vi "Initialize DAQDict Ref.vi"(8 "error in (no error)":errorcluster) -> (0 "error out":errorcluster, 3 "dCVT DAQDict out":T1)   [LabVIEW 2020, in "DAQDict.lvlib"]
uses:
  DAQDict.lvlib
  <vilib>/TELLC/Dynamic CVT API/TD Dynamic CVT DVR--ref.ctl
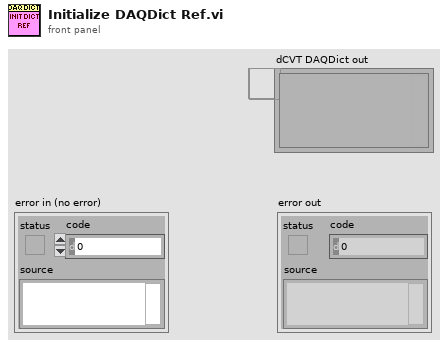
[diagram p1: front panel]
types:
  T1 = typedef "TD Dynamic CVT DVR--ref.ctl" = refnum<data-value>
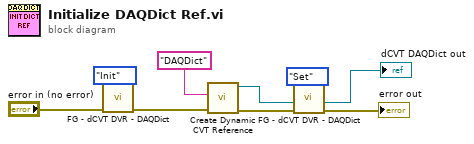
[diagram p0: block diagram]
diagram:
  n1 = call "FG - dCVT DVR - DAQDict.vi"("error in (no error)"="error in (no error)", "Action (Get)"=enum16{"Init", "Get", "Set"}."Init") -> ("error out"=w6:errorcluster)  [unwired: 7 in, 1 out]
  n2 = call <vilib>:"Create Dynamic CVT Reference.vi"("error in (no error)"=w6, "DictName"="DAQDict") -> ("error out"=w9:errorcluster, "dCVT DVR out"=w2:T1)  [unwired: 8 in]
  n3 = call "FG - dCVT DVR - DAQDict.vi"("dCVT DAQDict"=w2, "error in (no error)"=w9, "Action (Get)"=enum16{"Init", "Get", "Set"}."Set") -> ("dCVT DAQDict out"=→"dCVT DAQDict out":T1, "error out"=→"error out":errorcluster)  [unwired: 6 in]
